vi "WheelShooter Master.vi"(1 "input cluster":T1) -> (0 "error out":errorcluster)   [LabVIEW 2015]
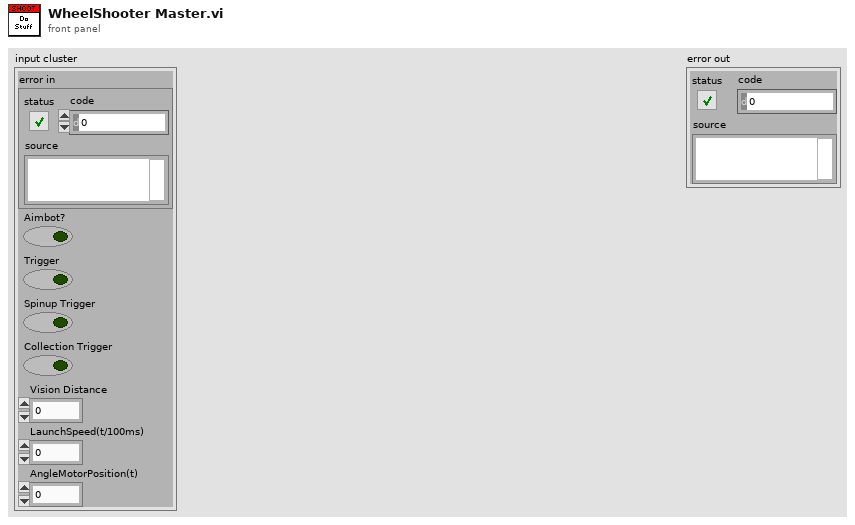
[diagram p1: front panel]
types:
  T1 = cluster{"error in":errorcluster, "Aimbot?":bool, "Trigger":bool, "Spinup Trigger":bool, "Collection Trigger":bool, "Vision Distance":dbl, "LaunchSpeed(t/100ms)":dbl, "AngleMotorPosition(t)":dbl}
  T2 = typedef "WPI_MotorControlDeviceRef.ctl" = cluster{"DeviceStatus":errorcluster, "Type":T3, "PWM":cluster{"PWM Channel":T4, "DeadBand":T5}, "CAN":cluster{"Device Number":u8, "Control Mode":T6, "Semaphore":T7, "Max Vout":dbl, "TalonSRX Control Mode":T8}, "Invert":bool}
  T3 = typedef "WPI_MotorControlType.ctl" = enum16{"PWM", "CAN", "CANTalonSRX"}
  T4 = typedef "FPGA_DIOPWMChannel.ctl" = enum8{"PWM 0", "PWM 1", "PWM 2", "PWM 3", "PWM 4", "PWM 5", "PWM 6", "PWM 7", "PWM 8", "PWM 9", "PWM MXP 0", "PWM MXP 1", "PWM MXP 2", "PWM MXP 3", "PWM MXP 4", "PWM MXP 5", "PWM MXP 6", "PWM MXP 7", "PWM MXP 8", "PWM MXP 9", "Invalid"}
  T5 = typedef "WPI_PWMDeadband.ctl" = cluster{"Name":string, "maxPositivePwm":i32, "minPositivePwm":i32, "centerPwm":i32, "maxNegativePwm":i32, "minNegativePwm":i32, "angularRange":u16}
  T6 = typedef "WPI_CANJaguar_ControlMode.ctl" = enum8{"Percent VBus", "Current", "Speed", "Position", "Voltage"}
  T7 = typedef "Semaphore RefNum" = refnum<k1>
  T8 = typedef "WPI_CANTalonSRX_APIControlMode.ctl" = enum8{"Percent VBus", "Speed", "Position", "Slave", "Unchanged / Invalid", "Voltage Compensation", "Current", "Motion Profile"}
  T9 = typedef "WPI_ServoDeviceRef.ctl" = cluster{"DeviceStatus":errorcluster, "PWM Channel":T4, "DeadBand":T5}
  T10 = cluster{"error":errorcluster, "AngleMotorRefnum":T2, "LeftWheelRefnum":T2, "RightWheelRefnum":T2, "PushServoRefnum":T9, "AngleMotorPosition(t)":dbl, "LaunchSpeed(t/100ms)":dbl, "CollectSpeed(t/100ms)":dbl, "SpinUpDuration(10ms)":i32, "ShotDuration(10ms)":i32, "PushServoAngle":i32}
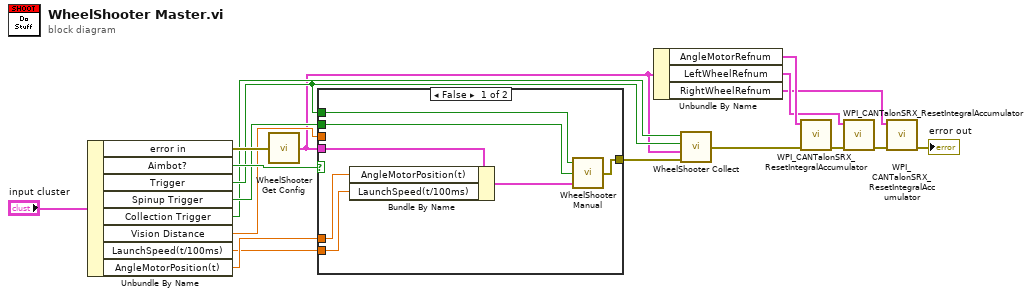
[diagram p0: block diagram]
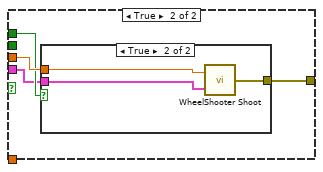
[diagram p2: hidden frame]
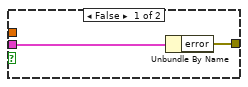
[diagram p3: hidden frame]
diagram:
  n1 = Unbundle By Name("input cluster") -> ("error in"=w17:errorcluster, "Aimbot?"=w16:bool, "Trigger"=w15:bool, "Spinup Trigger"=w14:bool, "Collection Trigger"=w13:bool, "Vision Distance"=w12:dbl, "LaunchSpeed(t/100ms)"=w10:dbl, "AngleMotorPosition(t)"=w11:dbl)
  n2 = call "WheelShooter Get Config.vi"("error in"=w17) -> ("cluster out"=w4:T10)
  n3 = case shown="False" w16 {
    tunnel: w12 -> [_ w29]
    tunnel: w15 -> [w25 w28]
    tunnel: w14 -> [w24 _]
    tunnel: w4 -> [w21 w27]
    tunnel: w11 -> [w23 _]
    tunnel: w10 -> [w22 _]
    tunnel: [w20 w26] -> w18
    frame False {
      n4 = Bundle By Name(cluster=w21, "AngleMotorPosition(t)"=w23, "LaunchSpeed(t/100ms)"=w22) -> (w19:T10)
      n5 = call "WheelShooter Manual.vi"("cluster in"=w19, "Spinup Trigger"=w24, "Trigger"=w25) -> ("error out"=w20:errorcluster)
    }
    frame True {
      n6 = case shown="True" w28 {
        tunnel: w29 -> [_ w34]
        tunnel: w27 -> [w31 w33]
        tunnel: [w30 w32] -> w26
        frame False {
          n7 = Unbundle By Name(w31) -> ("error"=w30:errorcluster)
        }
        frame True {
          n8 = call "WheelShooter Shoot.vi"("cluster in"=w33, "Range"=w34) -> ("error out"=w32:errorcluster)
        }
      }
    }
  }
  n9 = Unbundle By Name(w4) -> ("AngleMotorRefnum"=w3:T2, "LeftWheelRefnum"=w2:T2, "RightWheelRefnum"=w1:T2)
  n10 = call "WheelShooter Collect.vi"("error in (no error)"=w18, "cluster in"=w4, "Trigger"=w15, "CollectionTrigger"=w13) -> ("error out"=w6:errorcluster)
  n11 = call <vilib>:"WPI_CANTalonSRX_ResetIntegralAccumulator.vi"("error in (no error)"=w6, "CAN Talon SRX Ref"=w3) -> ("error out"=w7:errorcluster)  [unwired: 8 in, 1 out]
  n12 = call <vilib>:"WPI_CANTalonSRX_ResetIntegralAccumulator.vi"("error in (no error)"=w7, "CAN Talon SRX Ref"=w2) -> ("error out"=w8:errorcluster)  [unwired: 8 in, 1 out]
  n13 = call <vilib>:"WPI_CANTalonSRX_ResetIntegralAccumulator.vi"("error in (no error)"=w8, "CAN Talon SRX Ref"=w1) -> ("error out"=→"error out":errorcluster)  [unwired: 8 in, 1 out]
